vi "string to bool small.vi"(7 "String":string) -> (8 "number":bool)   [LabVIEW 2018]
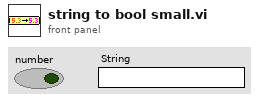
[diagram p1: front panel]
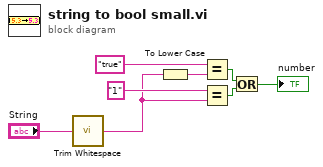
[diagram p0: block diagram]
diagram:
  n1 = call <vilib>:"Trim Whitespace.vi"("string"="String") -> ("trimmed string"=w1:string)  [unwired: 1 in]
  n2 = To Lower Case(string=w1) -> (all lower case string=w7:string)
  n3 = Equal?(x="true", y=w7) -> (x = y?=w4:bool)
  n4 = Equal?(x="1", y=w1) -> (x = y?=w5:bool)
  n5 = Or(x=w4, y=w5) -> (x .or. y?=→"number":bool)
